vi "ui-form-text-line.vi"(11 "User Prompt in":string) -> (1 "Cancelled?":bool, 2 "text out":string)   [LabVIEW 2024]
doc: "Use this template to build a user interface event handler design pattern. Use this pattern for dialog boxes and other user interfaces. You also can create and execute user-defined events that the VI can handle the same way as user interface events."
uses:
  <vilib>/Utility/miscctls.llb/LVPointTypeDef.ctl
panel:
  in  "User Input":string
  in  "Cancel Button":bool
  in  "OK Button":bool
  in  "stop":bool
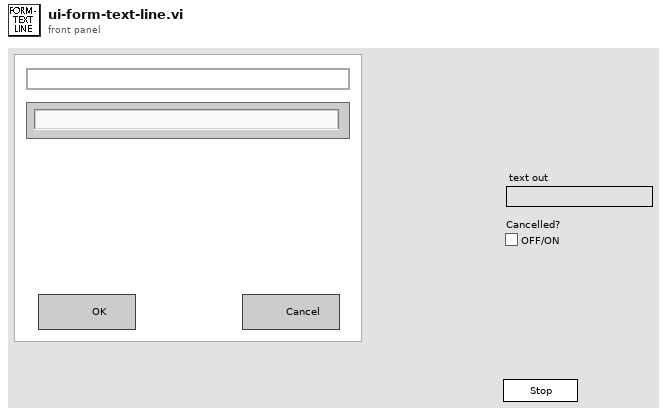
[diagram p1: front panel]
types:
  T1 = typedef "LVPointTypeDef.ctl" = cluster{"Horizontal":i16, "Vertical":i16}
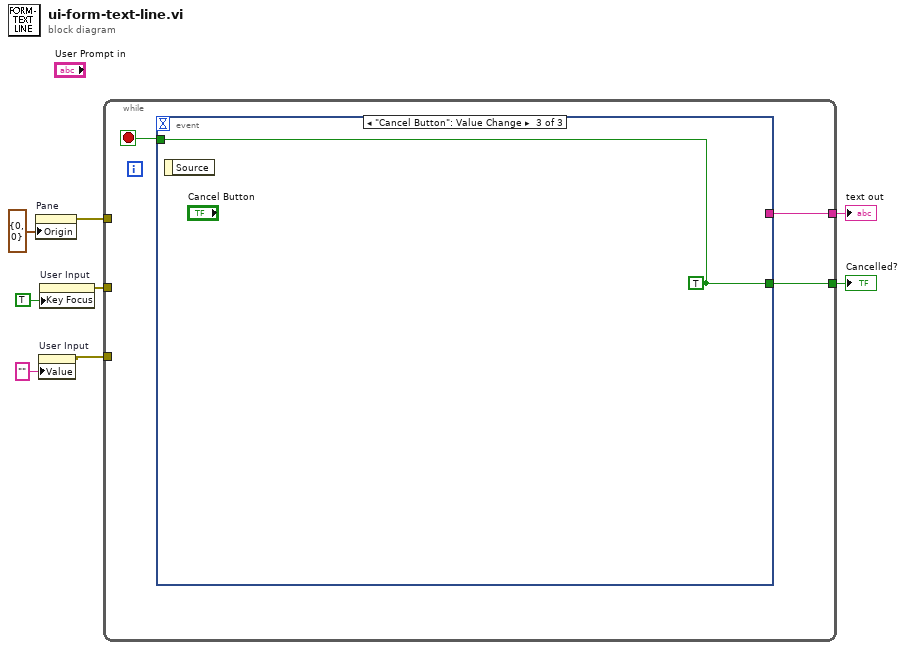
[diagram p0: block diagram]
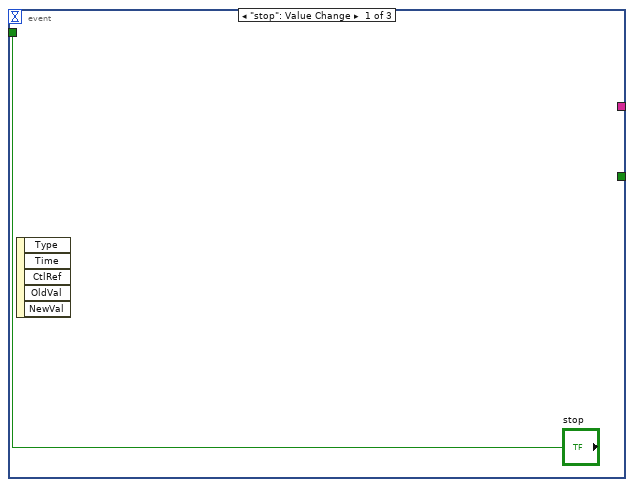
[diagram p2: hidden frame]
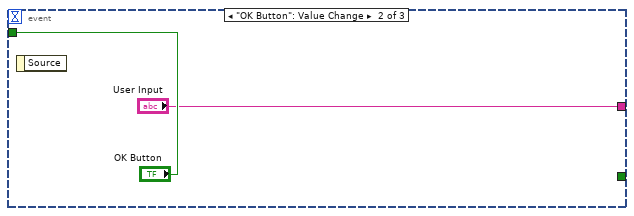
[diagram p3: hidden frame]
diagram:
  n1 = property on="Pane" class="Pane"("Origin"=T1 {"Horizontal"=0, "Vertical"=0}) -> (error out=w4:errorcluster)  [unwired: 2 in, 1 out]
  n2 = property on="User Input" class="Str"("Value"="" ("User Input")) -> (error out=w2:errorcluster)  [unwired: 2 in, 1 out]
  n3 = property on="User Input" class="Str"("Key Focus"=TRUE) -> (error out=w5:errorcluster)  [unwired: 2 in, 1 out]
  n4 = while {
    tunnel: [w10] -> w8
    tunnel: [w9] -> w7
    tunnel: w5 -> [_]
    tunnel: w4 -> [_]
    tunnel: w2 -> [_]
    stop <- w11 stop-if-true
    n5 = event shown="[2] \"Cancel Button\": Value Change" {
      selector: _ -> [_ _ _]
      dyn-events: _ -> [_ _ _]
      timeout: _ -> [_ _ _]
      tunnel: ["stop" "OK Button" w15] -> w11
      tunnel: [_ _ w15] -> w10
      tunnel: [_ "User Input" _] -> w9
      event "stop": Value Change {
        n6 = event-data() -> ()  [unwired: 1 in, 5 out]
      }
      event "OK Button": Value Change {
        n7 = event-data() -> ()  [unwired: 1 in, 1 out]
      }
      event "Cancel Button": Value Change {
        w15 = TRUE ("OK Button")
        n8 = event-data() -> ()  [unwired: 1 in, 1 out]
      }
    }
  }
  "Cancelled?" <- w8
  "text out" <- w7
